vi "DBCisMutiplex.vi"(11 "Sg":string) -> (3 "Style10":string)   [LabVIEW 2015]
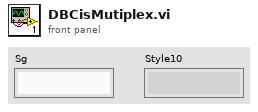
[diagram p1: front panel]
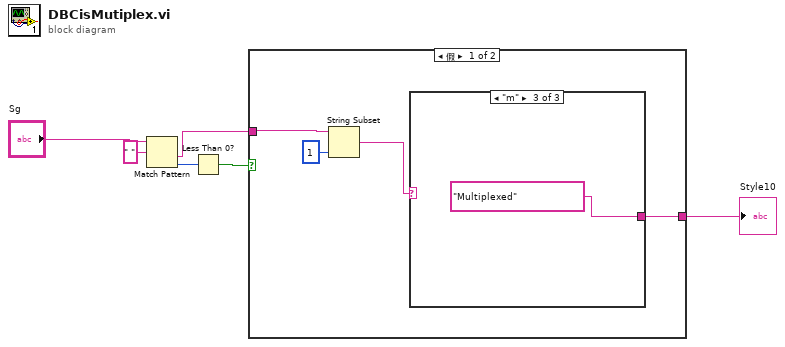
[diagram p0: block diagram]
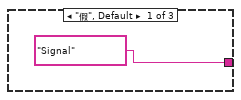
[diagram p2: hidden frame]
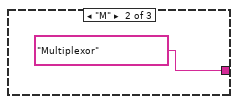
[diagram p3: hidden frame]
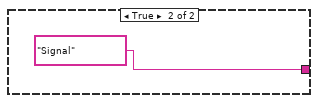
[diagram p4: hidden frame]
diagram:
  n1 = Match Pattern(string="Sg", regular expression=" " ("正则表达式")) -> (after substring=w1:string, offset past match=w2:i32)  [unwired: 1 in, 2 out]
  n2 = Less Than 0?(x=w2) -> (x < 0?=w4:bool)
  n3 = case shown="假" w4 {
    tunnel: [w7 "Signal"] -> w3
    tunnel: w1 -> [w10 _]
    frame False {
      n4 = String Subset(string=w10, length (rest)=1 ("长度（剩余）")) -> (substring=w8:string)  [unwired: 1 in]
      n5 = case shown="\"m\"" w8 {
        tunnel: ["Signal" "Multiplexor" "Multiplexed"] -> w7
        frame "假", Default {
        }
        frame "M" {
        }
        frame "m" {
        }
      }
    }
    frame True {
    }
  }
  "Style10" <- w3
